vi "tiffClose.vi"(11 "Tiff in":refnum<k24>) -> (3 "FileName":string)   [LabVIEW 2012, in "LVTiffWriter.lvlib"]
doc: "Finishes file writing and closes it."
uses:
  LVTiffWriter.lvlib
  D:/MyDocuments/LabVIEW Data/SPIM/LVTiffWriter/libtiff.net_bin-2.4.500.0/BitMiracle.LibTiff.NET.dll
  BitMiracle.LibTiff.NET.dll
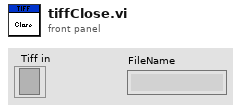
[diagram p1: front panel]
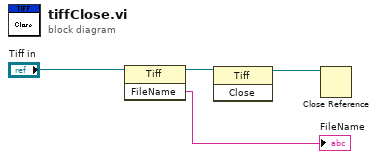
[diagram p0: block diagram]
diagram:
  n1 = invoke class="Tiff" method="FileName"(reference="Tiff in") -> (reference out=w3:refnum<k24>, "FileName"=→"FileName":string)  [unwired: 2 in, 1 out]
  n2 = invoke class="Tiff" method="Close"(reference=w3) -> (reference out=w4:refnum<k24>)  [unwired: 2 in, 2 out]
  n3 = Close Reference(reference=w4) -> ()  [unwired: 1 in, 1 out]
